vi "ErrorClusterExample.vi"() -> ()   [LabVIEW 2019]
panel:
  out "remaining string":string
  out "Error Out":errorcluster
  in  "Error In":errorcluster
  in  "Input data":string="Hello I am Atharva, I live in Nagpur and i am 21 years old"
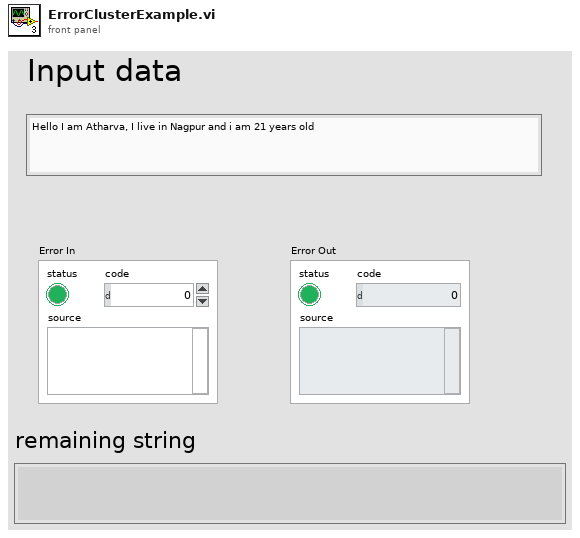
[diagram p1: front panel]
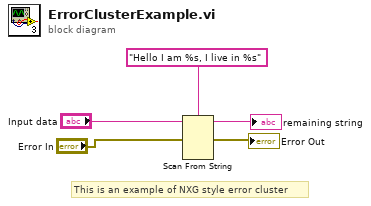
[diagram p0: block diagram]
diagram:
  # "This is an example of NXG style error cluster"
  n1 = Scan From String(format string="Hello I am %s, I live in %s", input string="Input data", error in="Error In") -> (remaining string=→"remaining string":string, error out=→"Error Out":errorcluster)  [unwired: 5 in, 1 out]
